vi "QTMDriver.vi"(0 "connection ID":refnum<k5>, 1 "Ring":T1, 5 "DataIn":dbl[](array[numeric]), 7 "QTMqueue":refnum<queue>, 9 "VI Refnum QTMTask":refnum<vi>, 11 "error in":errorcluster, 12 "timeout ms (25000)":i32=6000, 13 "DataOutIndex":i32=1) -> (3 "ArrayOut":dbl[](array[numeric]), 4 "connection ID out":refnum<k5>, 6 "DataOut":dbl[](array[numeric]), 8 "QTMqueue Out":refnum<queue>, 10 "return count":u32, 14 "VI Refnum QTMTask Out":refnum<vi>, 15 "error out":errorcluster)   [LabVIEW 2010]
uses:
  CustomIO.ctl
  <vilib>/Instr/_visa.llb/VISA Configure Serial Port (Instr).vi
panel:
  in  "flow control":u32(ring) items=["None", "XON/XOFF", "RTS/CTS", "XON/XOFF & RTS/CTS", "DTR/DSR", "XON/XOFF & DTR/DSR"]
  in  "stop bits":u32(ring)=10 items=["1.0"=10, "1.5"=15, "2.0"=20]
  in  "parity":enum32{"None", "Odd", "Even", "Mark", "Space"}(ring)=enum."Even"
  in  "data bits":u32=8
  in  "baud rate":u32=115200
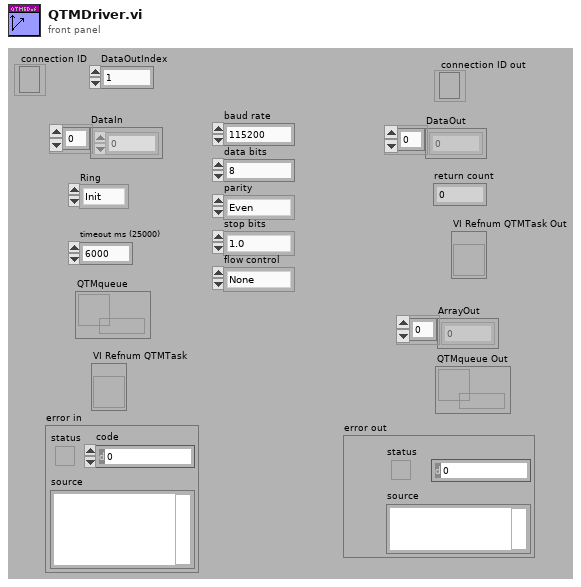
[diagram p1: front panel]
types:
  T1 = typedef "CustomIO.ctl" = enum16{"Init", "Read", "Write", "Close", "N/O"}
  T2 = enum16{"big-endian, network order", "native, host order", "little-endian"}
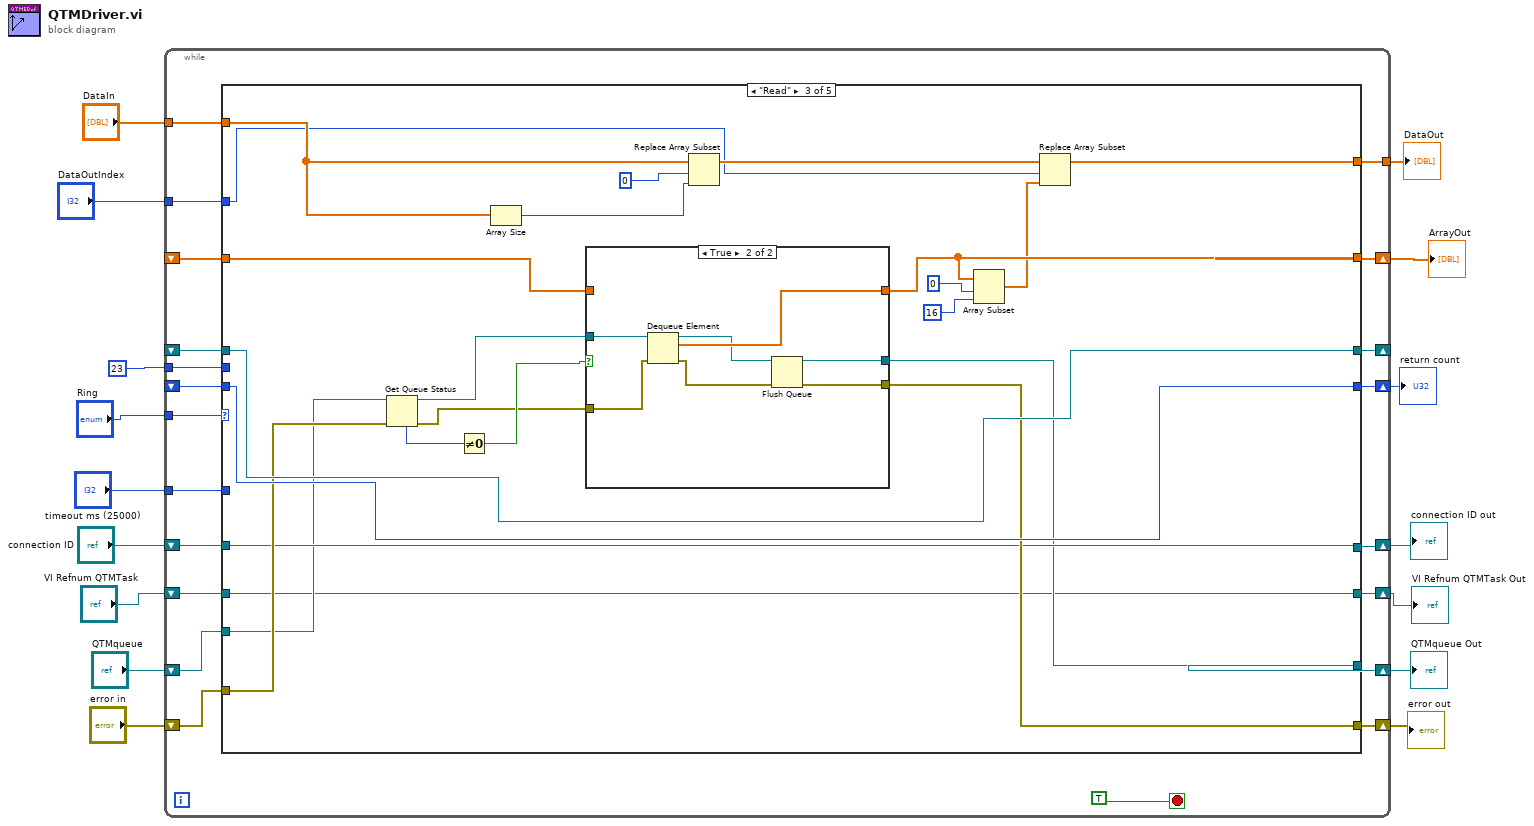
[diagram p0: block diagram]
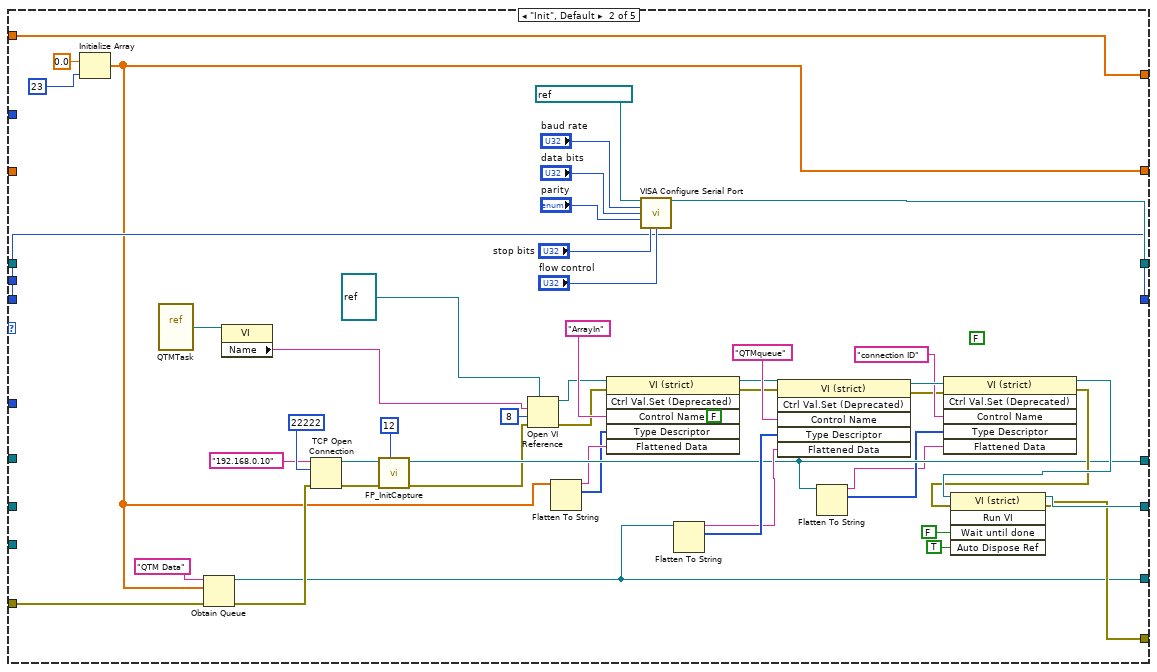
[diagram p3: hidden frame]
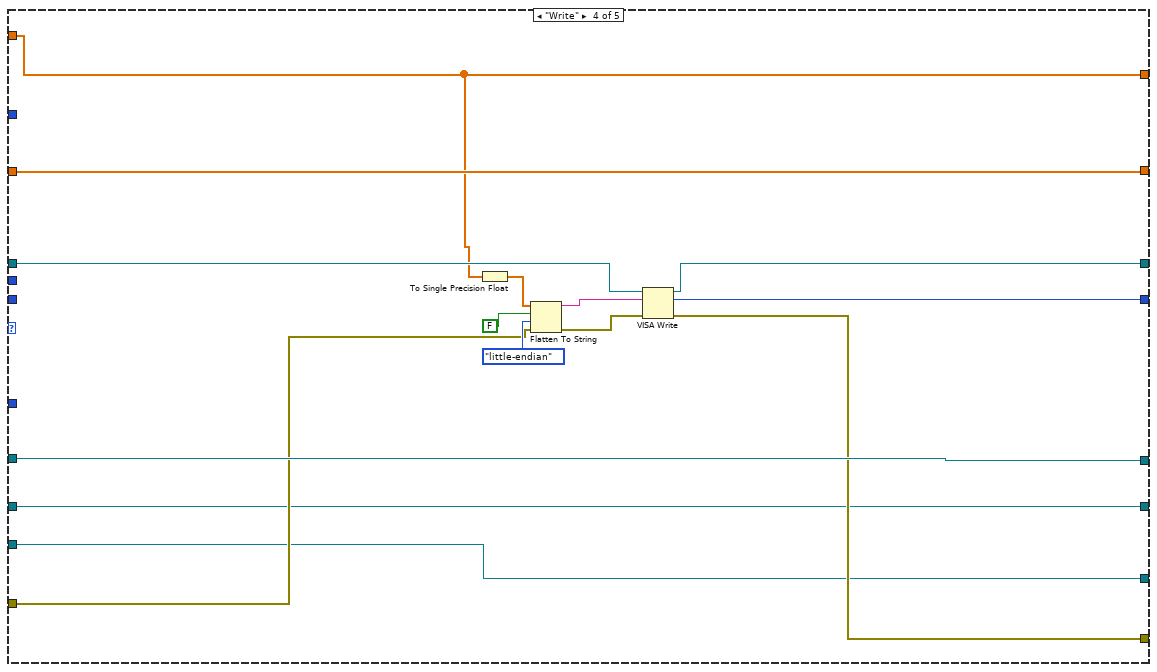
[diagram p5: hidden frame]
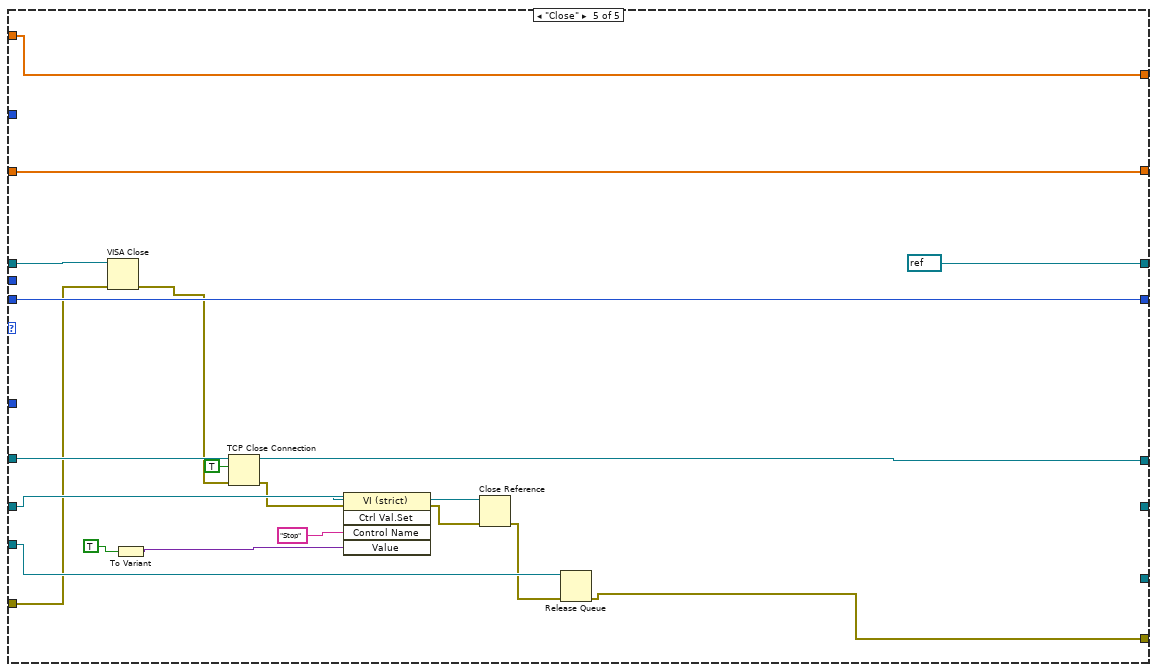
[diagram p6: hidden frame]
diagram:
  n1 = while {
    tunnel: "Ring" -> [w37]
    shift-right: [w36] -> w6
    shift-left: _ -> [w35]
    tunnel: 23 -> [w34]
    shift-right: [w32] -> w14
    shift-left: "error in" -> [w33]
    shift-right: [w30] -> w12
    shift-left: "connection ID" -> [w31]
    tunnel: "DataIn" -> [w29]
    tunnel: [w28] -> w10
    tunnel: "DataOutIndex" -> [w27]
    tunnel: "timeout ms (25000)" -> [w26]
    shift-right: [w25] -> _
    shift-left: _ -> [w24]
    shift-right: [w23] -> w7
    shift-left: _ -> [w22]
    shift-right: [w21] -> w3
    shift-left: "QTMqueue" -> [w20]
    shift-right: [w19] -> w1
    shift-left: "VI Refnum QTMTask" -> [w18]
    stop <- TRUE stop-if-true
    n2 = case shown="\"Read\"" w37 {
      tunnel: [w45 w51 w95 w135 w158] -> w36
      tunnel: w35 -> [w45 _ w105 w135 w158]
      tunnel: w34 -> [_ _ _ _ _]
      tunnel: w33 -> [w44 w76 w108 w132 w150]
      tunnel: [w44 w69 w102 w131 w149] -> w32
      tunnel: w31 -> [w38 _ w101 w141 w160]
      tunnel: [w38 w58 w101 w141 w159] -> w30
      tunnel: w29 -> [w43 w89 w113 w129 w157]
      tunnel: [w43 w89 w112 w129 w157] -> w28
      tunnel: w27 -> [_ _ w111 _ _]
      tunnel: w26 -> [_ _ _ _ _]
      tunnel: [w42 w81 w110 w133 refnum<visa-resource-name> refnum ("VISA resource name out")] -> w25
      tunnel: w24 -> [w42 _ w110 w134 w156]
      tunnel: [w41 w80 w109 w130 w154] -> w23
      tunnel: w22 -> [w41 w80 w109 _ w154]
      tunnel: [w40 w68 w99 w128 _] -> w21
      tunnel: w20 -> [w40 _ w100 w128 w152]
      tunnel: [w39 w71 w98 w127 _] -> w19
      tunnel: w18 -> [w39 _ w98 w127 w153]
      frame "N/O" {
      }
      frame "Init", Default {
        (unwired) FALSE ("Wait Until Done")
        (unwired) FALSE ("Stop")
        n3 = Initialize Array(0.0 ("element"), 23) -> (w51:dbl[])
        n4 = vi-ref "QTMTask.vi"() -> (w72:refnum<vi>)
        n5 = Obtain Queue(name (unnamed)="QTM Data", element data type=w51, error in (no error)=w76) -> (queue out=w68:refnum<queue>, error out=w75:errorcluster)  [unwired: 2 in, 1 out]
        n6 = property class="VI"(reference=w72) -> ("Name"=w54:string)  [unwired: 1 in, 2 out]
        n7 = TCP Open Connection(address="192.168.0.10", remote port or service name=u16 22222, error in (no error)=w75) -> (connection ID=w93:refnum<k5>, error out=w92:errorcluster)  [unwired: 2 in]
        n8 = call "FP_InitCapture.vi"("ComponentType"=u32 12, "error out 2"=w92, "connection ID"=w93) -> ("error out"=w55:errorcluster, "connection ID out"=w58:refnum<k5>)  [unwired: 5 in, 2 out]
        n9 = Open VI Reference(type specifier VI Refnum (for type only)=refnum<vi> refnum, vi path=w54, options=8, error in (no error)=w55) -> (vi reference=w47:refnum<vi>, error out=w46:errorcluster)  [unwired: 2 in]
        n10 = Flatten To String(anything=w51) -> (data string=w50:string, type string=w49:i16[])  [unwired: 1 in, 3 out]
        n11 = invoke class="VI (strict)" method="Ctrl Val.Set (Deprecated)"(reference=w47, error in=w46, "Control Name"="ArrayIn", "Type Descriptor"=w49, "Flattened Data"=w50) -> (reference out=w53:refnum<vi>, error out=w52:errorcluster)  [unwired: 1 in, 4 out]
        n12 = call-poly "VISA Configure Serial Port"("VISA resource name"=refnum<visa-resource-name> "ASRL1::INSTR", "baud rate (9600)"="baud rate", "data bits (8)"="data bits", "parity (0:none)"="parity", "stop bits (10: 1 bit)"="stop bits", "flow control (0:none)"="flow control") -> ("VISA resource name out"=w81:refnum<visa-resource-name>)  [unwired: 1 in, 8 out]
        n13 = Flatten To String(anything=w68) -> (data string=w60:string, type string=w61:i16[])  [unwired: 1 in, 3 out]
        n14 = invoke class="VI (strict)" method="Ctrl Val.Set (Deprecated)"(reference=w53, error in=w52, "Control Name"="QTMqueue", "Type Descriptor"=w61, "Flattened Data"=w60) -> (reference out=w67:refnum<vi>, error out=w64:errorcluster)  [unwired: 1 in, 4 out]
        n15 = Flatten To String(anything=w58) -> (data string=w56:string, type string=w57:i16[])  [unwired: 1 in, 3 out]
        n16 = invoke class="VI (strict)" method="Ctrl Val.Set (Deprecated)"(reference=w67, error in=w64, "Control Name"="connection ID", "Type Descriptor"=w57, "Flattened Data"=w56) -> (reference out=w65:refnum<vi>, error out=w63:errorcluster)  [unwired: 1 in, 4 out]
        n17 = invoke class="VI (strict)" method="Run VI"(reference=w65, error in=w63, "Wait until done"=FALSE ("Wait Until Done"), "Auto Dispose Ref"=TRUE ("Auto Dispose Reference")) -> (reference out=w71:refnum<vi>, error out=w69:errorcluster)  [unwired: 1 in, 3 out]
      }
      frame "Read" {
        n18 = Get Queue Status(queue=w100, error in (no error)=w108) -> (queue out=w104:refnum<queue>, error out=w103:errorcluster, # elements in queue=w107:i32)  [unwired: 1 in, 5 out]
        n19 = Not Equal To 0?(x=w107) -> (x != 0?=w106:bool)
        n20 = Array Size(array=w113) -> (size(s)=w114:i32)
        n21 = case shown="True" w106 {
          tunnel: w105 -> [w119 _]
          tunnel: w104 -> [w117 w126]
          tunnel: [w119 w125] -> w95
          tunnel: w103 -> [w118 w122]
          tunnel: [w118 w121] -> w102
          tunnel: [w117 w120] -> w99
          frame False {
          }
          frame True {
            n22 = Dequeue Element(queue=w126, error in (no error)=w122) -> (queue out=w124:refnum<queue>, element=w125:dbl[], error out=w123:errorcluster)  [unwired: 1 in, 1 out]
            n23 = Flush Queue(queue=w124, error in (no error)=w123) -> (queue out=w120:refnum<queue>, error out=w121:errorcluster)  [unwired: 1 out]
          }
        }
        n24 = Replace Array Subset(array=w113, new element=w114, index=0) -> (w115:dbl[])
        n25 = Array Subset(array=w95, index=0, length=16) -> (w94:dbl[])
        n26 = Replace Array Subset(array=w115, new element=w94, index=w111) -> (w112:dbl[])
      }
      frame "Write" {
        n27 = To Single Precision Float(number=w129) -> (single precision float=w137:sgl[])
        n28 = Flatten To String(anything=w137, prepend array or string size? (T)=FALSE, byte order (0:big-endian, network order)=T2."little-endian", error in (no error)=w132) -> (data string=w136:string, error out=w138:errorcluster)  [unwired: 1 out]
        n29 = VISA Write(VISA resource name=w134, write buffer=w136, error in (no error)=w138) -> (VISA resource name out=w133:refnum<visa-resource-name>, return count=w130:u32, error out=w131:errorcluster)
      }
      frame "Close" {
        n30 = VISA Close(VISA resource name=w156, error in (no error)=w150) -> ()  [unwired: 1 out]
        n31 = To Variant(anything=TRUE) -> (Variant=w145:variant)
        n32 = TCP Close Connection(connection ID=w160, abort (F)=TRUE, error in (no error)=w150) -> (connection ID out=w159:refnum<k5>, error out=w143:errorcluster)
        n33 = invoke class="VI (strict)" method="Ctrl Val.Set"(reference=w153, error in=w143, "Control Name"="Stop", "Value"=w145) -> (reference out=w148:refnum<vi>, error out=w142:errorcluster)  [unwired: 1 in, 3 out]
        n34 = Close Reference(reference=w148, error in (no error)=w142) -> (error out=w151:errorcluster)
        n35 = Release Queue(queue=w152, error in (no error)=w151) -> (error out=w149:errorcluster)  [unwired: 1 in, 2 out]
      }
    }
  }
  "error out" <- w14
  "connection ID out" <- w12
  "DataOut" <- w10
  "return count" <- w7
  "ArrayOut" <- w6
  "QTMqueue Out" <- w3
  "VI Refnum QTMTask Out" <- w1
